vi "QTrkWaitForResults.vi"(10 "wanted results":i32, 11 "QTrk Instance":T1={"QTrk Pointer"=0, "QTrk Settings"={"Image width"=150, "Image height"=150, "Number of threads (CPU based)"=-1, "Max Queue Size"=128, "XCOR Profile Length"=32, "XCOR Profile Width"=2, "XCOR Iterations"=5, "ZLUT MinRadius"=50.0, "ZLUT MaxRadius"=64.0, "ZLUT AngularSteps"=0, "QI Iterations"=64, "QI RadialSteps"=64, "QI AngularSteps"=2, "QI MinRadius"=50.0, "QI MaxRadius"=50.0, "CUDA Device# (if using cuda)"=0}}) -> (3 "QTrk Instance (out)":T1={"QTrk Pointer"=0, "QTrk Settings"={"Image width"=150, "Image height"=150, "Number of threads (CPU based)"=-1, "Max Queue Size"=128, "XCOR Profile Length"=32, "XCOR Profile Width"=2, "XCOR Iterations"=5, "ZLUT MinRadius"=50.0, "ZLUT MaxRadius"=64.0, "ZLUT AngularSteps"=0, "QI Iterations"=64, "QI RadialSteps"=64, "QI AngularSteps"=2, "QI MinRadius"=50.0, "QI MaxRadius"=50.0, "CUDA Device# (if using cuda)"=0}})   [LabVIEW 2011]
uses:
  QTrkInstance.ctl
  QTrkSettings.ctl
panel:
  out "result count":i32
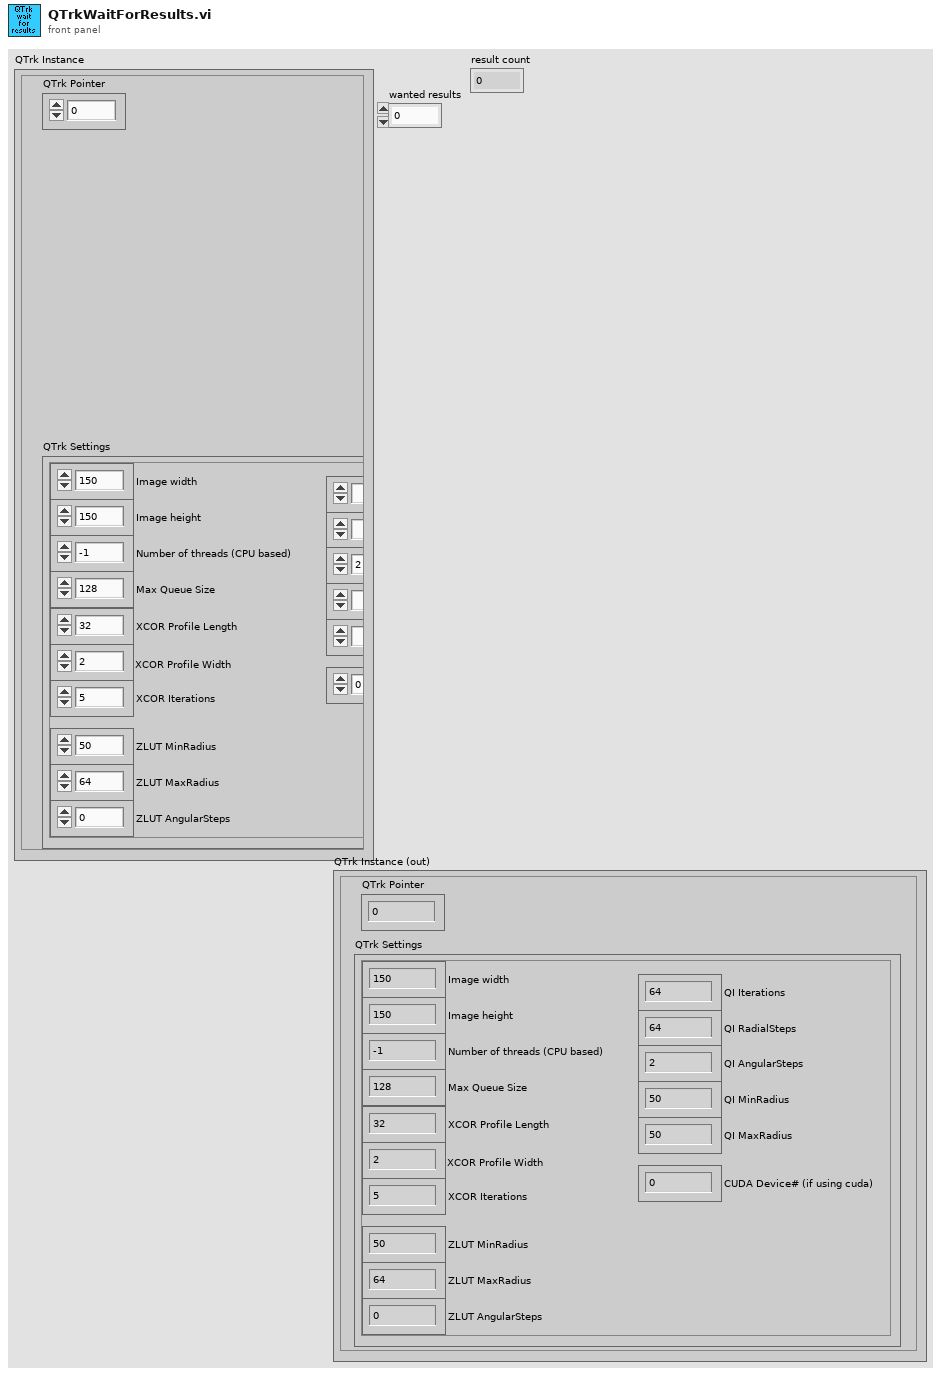
[diagram p1: front panel]
types:
  T1 = typedef "QTrkInstance.ctl" = cluster{"QTrk Pointer":u64, "QTrk Settings":T2}
  T2 = typedef "QTrkSettings.ctl" = cluster{"Image width":i32, "Image height":i32, "Number of threads (CPU based)":i32, "Max Queue Size":i32, "XCOR Profile Length":i32, "XCOR Profile Width":i32, "XCOR Iterations":i32, "ZLUT MinRadius":sgl, "ZLUT MaxRadius":sgl, "ZLUT AngularSteps":i32, "QI Iterations":i32, "QI RadialSteps":i32, "QI AngularSteps":i32, "QI MinRadius":sgl, "QI MaxRadius":sgl, "CUDA Device# (if using cuda)":i32}
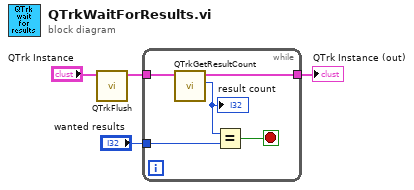
[diagram p0: block diagram]
diagram:
  n1 = call "QTrkFlush.vi"("QTrk Instance"="QTrk Instance") -> ("QTrk Instance (out)"=w3:T1)  [unwired: 10 in]
  n2 = while {
    tunnel: w3 -> [w9]
    tunnel: "wanted results" -> [w7]
    tunnel: [w5] -> w1
    stop <- w6 stop-if-true
    n3 = call "QTrkGetResultCount.vi"("QTrk Instance"=w9) -> ("result count"=w8:i32, "QTrk Instance"=w5:T1)  [unwired: 5 in]
    "result count" <- w8
    n4 = Equal?(x=w8, y=w7) -> (x = y?=w6:bool)
  }
  "QTrk Instance (out)" <- w1
